vi "Lechman_Host_A.vi"() -> ()   [LabVIEW 2019]
panel:
  in  "Wysłany sygnał":bool
  out "Bool":bool
  in  "stop":bool
  out "Waveform Graph":dbl[](graph)
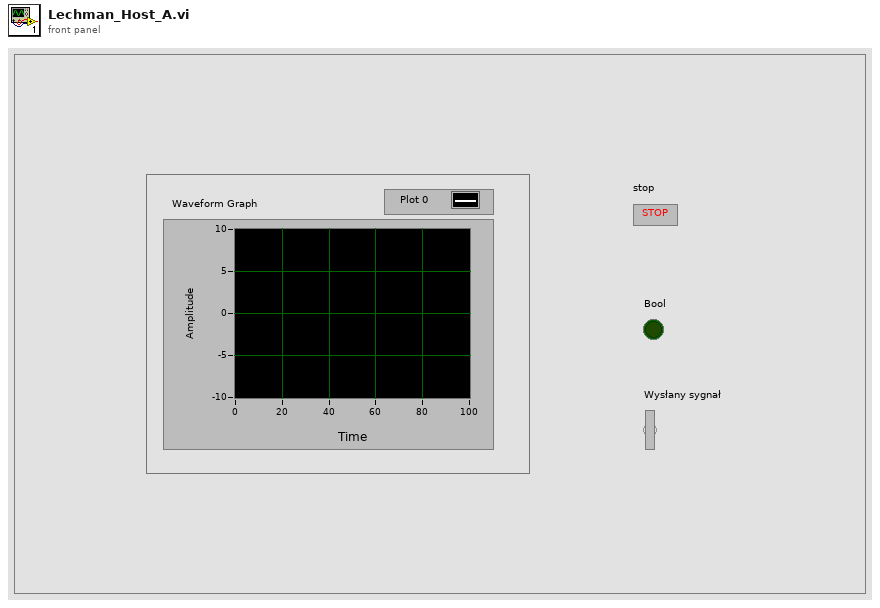
[diagram p1: front panel]
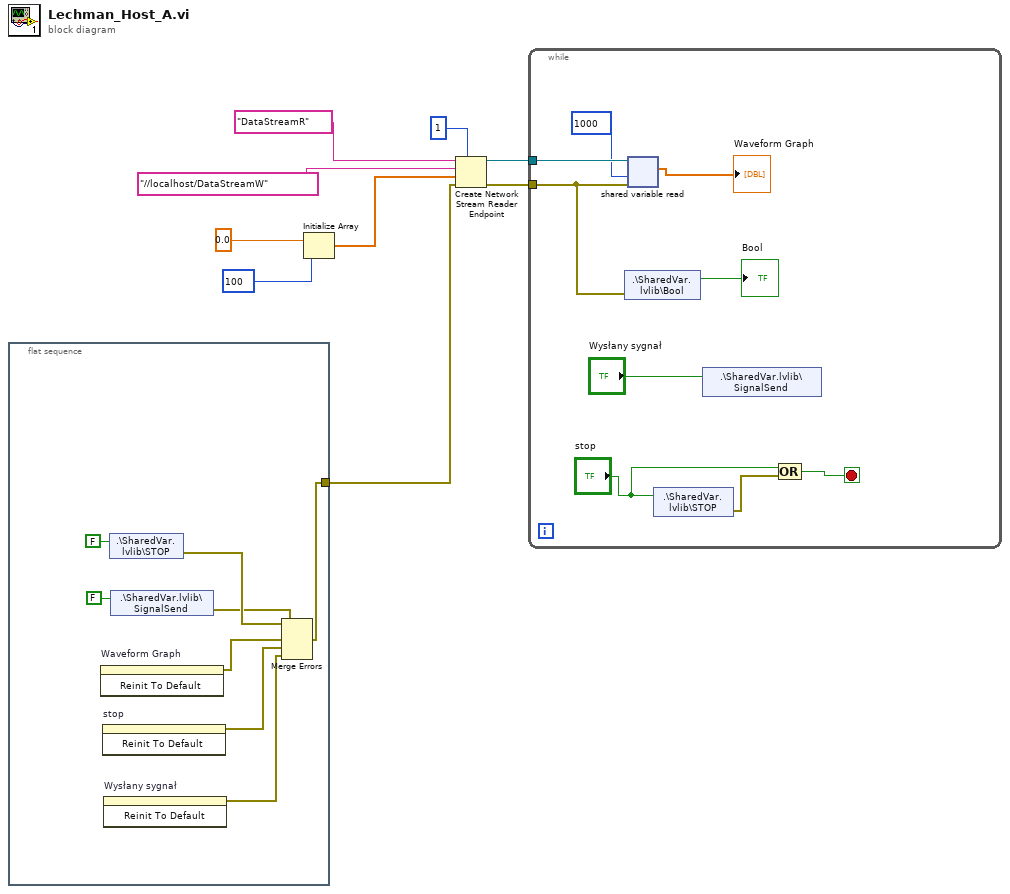
[diagram p0: block diagram]
diagram:
  n1 = flat-sequence {
    tunnel: [w10] -> w4
    frame #0 {
      n2 = invoke on="Waveform Graph" class="WFGraph (strict)" method="Reinit To Default"() -> (error out=w13:errorcluster)  [unwired: 3 in, 2 out]
      n3 = invoke on="stop" class="Bool" method="Reinit To Default"() -> (error out=w12:errorcluster)  [unwired: 3 in, 2 out]
      n4 = invoke on="Wysłany sygnał" class="Bool (strict)" method="Reinit To Default"() -> (error out=w11:errorcluster)  [unwired: 3 in, 2 out]
      n5 = shared-variable ".\\SharedVar.lvlib\\STOP"(FALSE ("STOP")) -> (error out=w15:errorcluster)  [unwired: 1 in]
      n6 = shared-variable ".\\SharedVar.lvlib\\SignalSend"(FALSE ("SignalSend")) -> (error out=w14:errorcluster)  [unwired: 1 in]
      n7 = Merge Errors(w15, w14, w13, w12, w11) -> (w10:errorcluster)
    }
  }
  n8 = Initialize Array(0.0, 100 ("dimension size")) -> (w5:dbl[])
  n9 = Create Network Stream Reader Endpoint(7:1 ("reader buffer size"), 8:w4, 9:w5, 10:"//localhost/DataStreamW" ("writer url"), 11:"DataStreamR" ("reader name")) -> (0:w3:errorcluster, 3:w2:refnum<k21>)  [unwired: 2 in]
  n10 = while {
    tunnel: w3 -> [w23]
    tunnel: w2 -> [w26]
    stop <- w19 stop-if-true
    n11 = shared-variable ".\\SharedVar.lvlib\\Bool"(error in=w23) -> (→"Bool":bool)  [unwired: 1 out]
    n12 = shared-variable-read(w26, w23, 1000 ("timeout ms (-1)")) -> (→"Waveform Graph":dbl[])  [unwired: 3 out]
    n13 = shared-variable ".\\SharedVar.lvlib\\STOP"("stop") -> (error out=w18:errorcluster)  [unwired: 1 in]
    n14 = shared-variable ".\\SharedVar.lvlib\\SignalSend"("Wysłany sygnał") -> ()  [unwired: 1 in, 1 out]
    n15 = Compound Arithmetic op=OR("stop", w18) -> (w19:bool)
  }
